vi "Calculate Step.vi"(9 "To":dbl, 10 "No of iterations":i32, 11 "From":dbl) -> (0 "error out":errorcluster, 3 "Step":dbl)   [LabVIEW 2020, in "Run Utilities.lvlib" / "Scan SBlock.lvclass"]
uses:
  Scan SBlock.lvclass
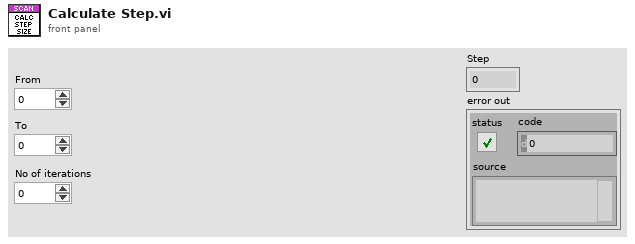
[diagram p1: front panel]
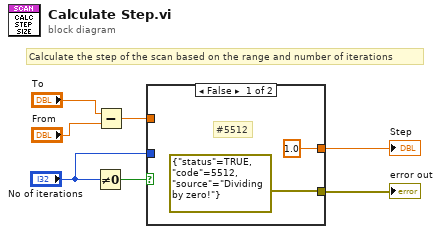
[diagram p0: block diagram]
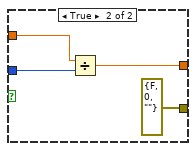
[diagram p2: hidden frame]
diagram:
  # "Calculate the step of the scan based on the range and number of iterations"
  n1 = Not Equal To 0?(x="No of iterations") -> (x != 0?=w7:bool)
  n2 = Subtract(x="To", y="From") -> (x-y=w6:dbl)
  n3 = case shown="False" w7 {
    tunnel: w6 -> [_ w13]
    tunnel: "No of iterations" -> [_ w12]
    tunnel: [1.0 w11] -> w4
    tunnel: [errorcluster {"status"=TRUE, "code"=5512, "source"="Dividing by zero!"} ("error out") errorcluster {"status"=FALSE, "code"=0, "source"=""} ("error out")] -> w3
    frame False {
      # "#5512"
    }
    frame True {
      n4 = Divide(x=w13, y=w12) -> (x/y=w11:dbl)
    }
  }
  "Step" <- w4
  "error out" <- w3
